vi "main.vi"() -> ()   [LabVIEW 2023]
uses:
  #typedef_typ.ctl
  #typedef_state.ctl
  #typdef_data.ctl
  08a89311-3c14-40fd-979e-0ee36f0e0fa9.vi
  <vilib>/Array/Sort 2D Array - Pop Stack.vi
  <vilib>/Array/Sort 2D Array - Push Stack.vi
  <vilib>/Utility/file.llb/Read Delimited Spreadsheet (string).vi
  <vilib>/Utility/file.llb/Write Delimited Spreadsheet (string).vi
panel:
  in  "Producent":string
  in  "Nazwa":string
  in  "Numer":string
  in  "Sort":bool
  in  "Add":bool
  in  "Delete":bool
  in  "Search":bool
  in  "Show":bool
  in  "Stop Button":bool
  in  "Produkt":string
  out "Wyswietlacz":string[][](array[string])
  in  "Type":T1
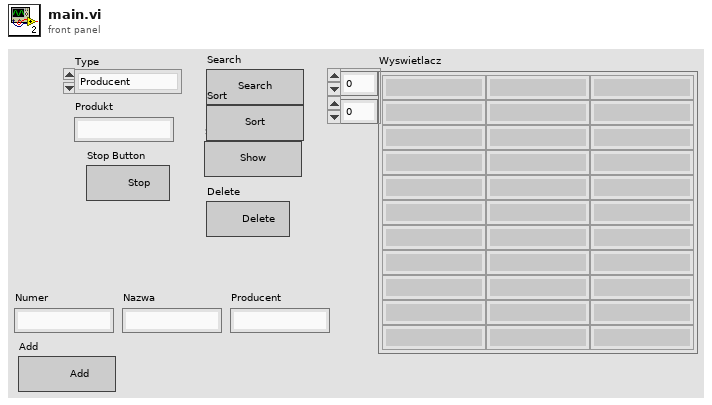
[diagram p1: front panel]
types:
  T1 = typedef "#typedef_typ.ctl" = enum16{"Producent", "Nazwa produktu", "Numer produktu"}
  T2 = typedef "#typedef_state.ctl" = enum16{"Aplication error", "Show", "Idle", "Open", "Search", "Add", "Delete", "Sort", "Exit"}
  T3 = typedef "#typdef_data.ctl" = cluster{"Type":enum16{"Producent", "Nazwa produktu", "Numer produktu"}, "Dane":string[][], "Produkt":string}
  T4 = enum16{"Producent", "Nazwa produktu", "Numer produktu"}
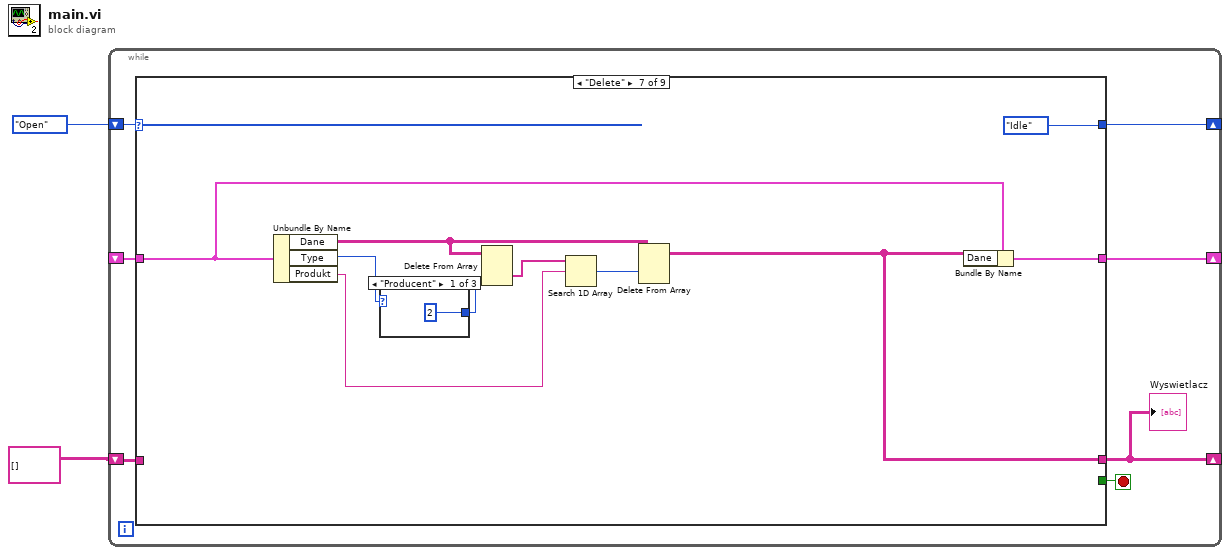
[diagram p0: block diagram]
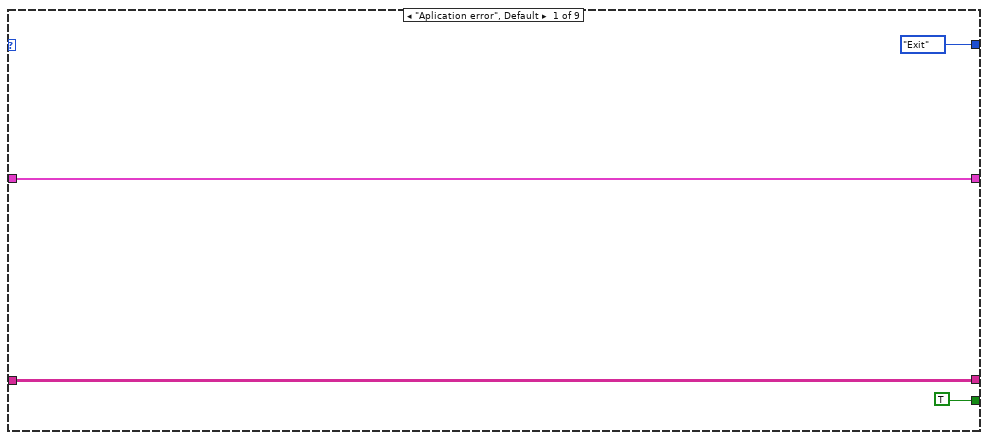
[diagram p2: hidden frame]
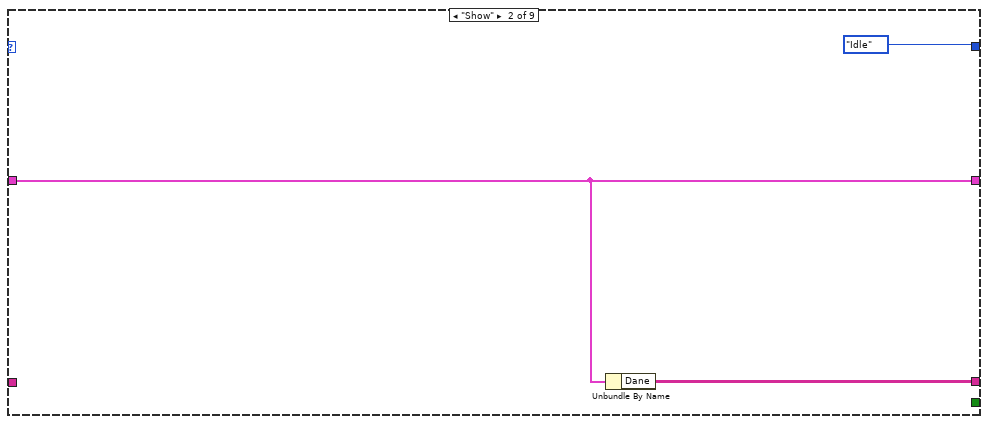
[diagram p3: hidden frame]
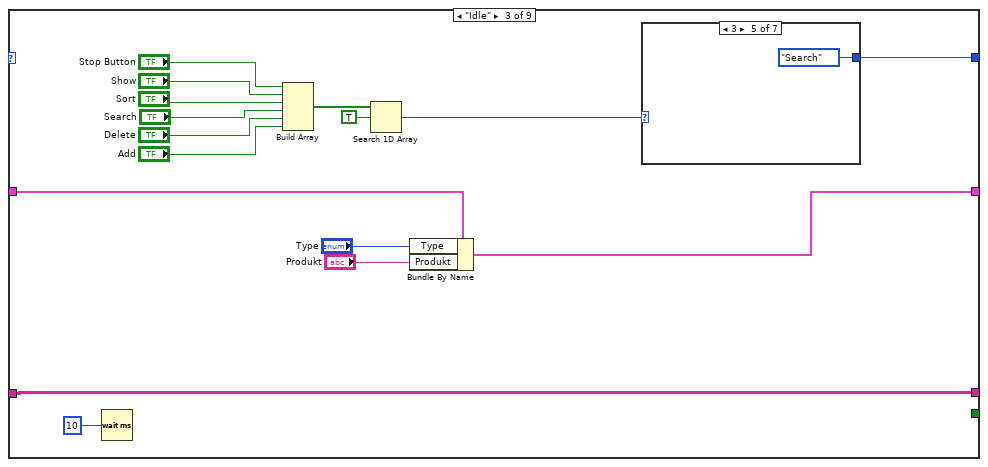
[diagram p4: hidden frame]
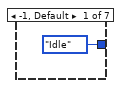
[diagram p5: hidden frame]
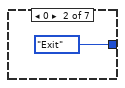
[diagram p6: hidden frame]
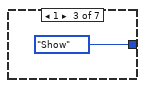
[diagram p7: hidden frame]
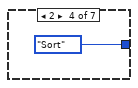
[diagram p8: hidden frame]
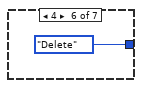
[diagram p9: hidden frame]
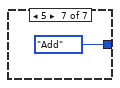
[diagram p10: hidden frame]
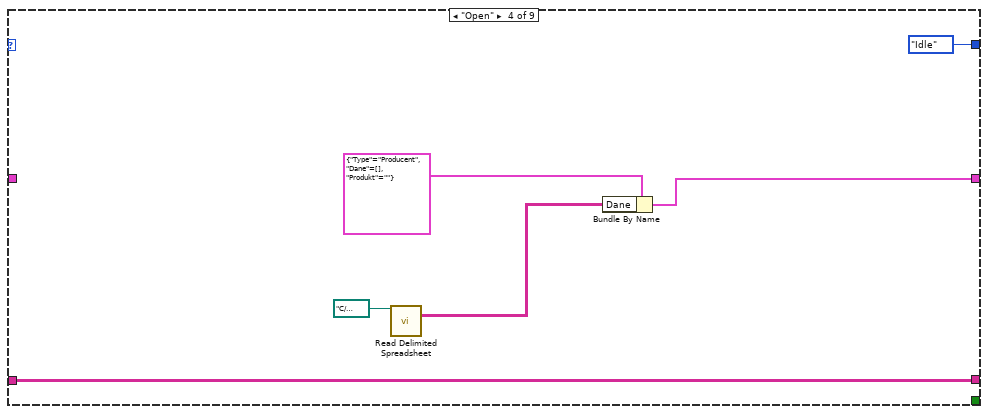
[diagram p11: hidden frame]
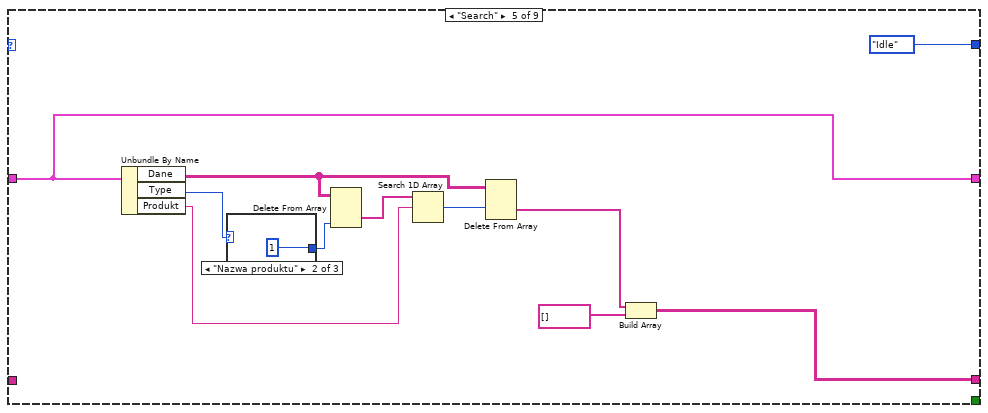
[diagram p12: hidden frame]
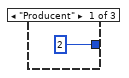
[diagram p13: hidden frame]
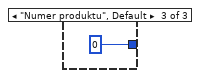
[diagram p14: hidden frame]
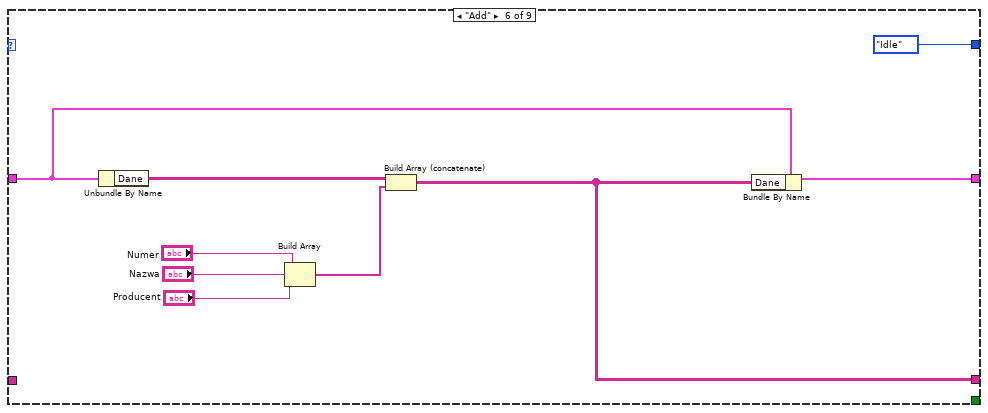
[diagram p15: hidden frame]
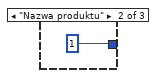
[diagram p16: hidden frame]
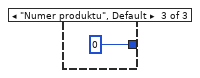
[diagram p17: hidden frame]
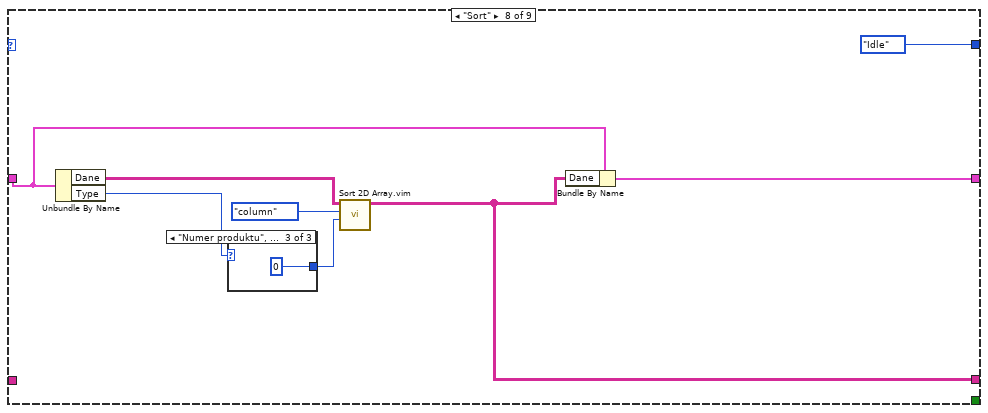
[diagram p18: hidden frame]
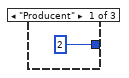
[diagram p19: hidden frame]
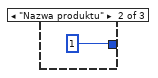
[diagram p20: hidden frame]
diagram:
  n1 = while {
    shift-right: [w8] -> _
    shift-left: #typedef_state."Open" ("State") -> [w9]
    shift-right: [w7] -> _
    shift-left: _ -> [w6]
    shift-right: [w3] -> _
    shift-left: string[][] [] ("Dane") -> [w4]
    stop <- w5 stop-if-true
    n2 = case shown="\"Delete\"" w9 {
      tunnel: [#typedef_state."Exit" ("State") #typedef_state."Idle" ("State") w17 #typedef_state."Idle" ("State") #typedef_state."Idle" ("State") #typedef_state."Idle" ("State") #typedef_state."Idle" ("State") #typedef_state."Idle" ("State") #typedef_state."Exit" ("State")] -> w8
      tunnel: [w12 w16 w28 w42 w50 w61 w73 w82 w96] -> w7
      tunnel: w6 -> [w12 w16 w32 _ w50 w63 w74 w83 w96]
      tunnel: [TRUE _ _ _ _ _ _ _ TRUE] -> w5
      tunnel: [w10 w15 w29 w40 w51 w62 w75 w84 w93] -> w3
      tunnel: w4 -> [w10 _ w29 w40 _ _ _ _ w93]
      frame "Aplication error", Default {
      }
      frame "Show" {
        n3 = Unbundle By Name(w16) -> ("Dane"=w15:string[][])
      }
      frame "Idle" {
        n4 = Wait (ms)(milliseconds to wait=u32 10) -> ()  [unwired: 1 out]
        n5 = Build Array("Stop Button", "Show", "Sort", "Search", "Delete", "Add") -> (w21:bool[])
        n6 = Search 1D Array(1D array=w21, element=TRUE) -> (index of element=w19:i32)  [unwired: 1 in]
        n7 = Bundle By Name(cluster=w32, "Type"="Type", "Produkt"="Produkt") -> (w28:T3)
        n8 = case shown="3" w19 {
          tunnel: [#typedef_state."Idle" ("State") #typedef_state."Exit" ("State") #typedef_state."Show" ("State") #typedef_state."Sort" ("State") #typedef_state."Search" ("State") #typedef_state."Delete" ("State") #typedef_state."Add" ("State")] -> w17
          frame -1, Default {
          }
          frame 0 {
          }
          frame 1 {
          }
          frame 2 {
          }
          frame 3 {
          }
          frame 4 {
          }
          frame 5 {
          }
        }
      }
      frame "Open" {
        n9 = call-poly <vilib>:"Read Delimited Spreadsheet.vi"("file path (dialog if empty)"=path "C:/Users/Python/Desktop/LabView Zadania/Wyklad - Maj/Zestaw 7 - State Machine/Zad2/baza.csv") -> ("all rows"=w41:string[][])  [unwired: 9 in, 5 out]
        n10 = Bundle By Name(cluster=T3 {"Type"=enum."Producent", "Dane"=[], "Produkt"=""} ("Data"), "Dane"=w41) -> (w42:T3)
      }
      frame "Search" {
        n11 = Unbundle By Name(w50) -> ("Dane"=w48:string[][], "Type"=w56:T4, "Produkt"=w55:string)
        n12 = case shown="\"Nazwa produktu\"" w56 {
          tunnel: [2 1 0] -> w47
          frame "Producent" {
          }
          frame "Nazwa produktu" {
          }
          frame "Numer produktu", Default {
          }
        }
        n13 = Delete From Array(array=w48, index (col)=w47) -> (deleted portion=w46:string[])  [unwired: 2 in, 1 out]
        n14 = Search 1D Array(1D array=w46, element=w55) -> (index of element=w54:i32)  [unwired: 1 in]
        n15 = Delete From Array(array=w48, index (row)=w54) -> (deleted portion=w53:string[])  [unwired: 2 in, 1 out]
        n16 = Build Array(w53, string[] [] ("element")) -> (w51:string[][])
      }
      frame "Add" {
        n17 = Unbundle By Name(w63) -> ("Dane"=w64:string[][])
        n18 = Build Array("Numer", "Nazwa", "Producent") -> (w65:string[])
        n19 = Build Array (concatenate)(w64, w65) -> (w62:string[][])
        n20 = Bundle By Name(cluster=w63, "Dane"=w62) -> (w61:T3)
      }
      frame "Delete" {
        n21 = Unbundle By Name(w74) -> ("Dane"=w71:string[][], "Type"=w78:T4, "Produkt"=w77:string)
        n22 = case shown="\"Producent\"" w78 {
          tunnel: [2 1 0] -> w70
          frame "Producent" {
          }
          frame "Nazwa produktu" {
          }
          frame "Numer produktu", Default {
          }
        }
        n23 = Delete From Array(array=w71, index (col)=w70) -> (deleted portion=w69:string[])  [unwired: 2 in, 1 out]
        n24 = Search 1D Array(1D array=w69, element=w77) -> (index of element=w76:i32)  [unwired: 1 in]
        n25 = Delete From Array(array=w71, index (row)=w76) -> (array with subset deleted=w75:string[][])  [unwired: 2 in, 1 out]
        n26 = Bundle By Name(cluster=w74, "Dane"=w75) -> (w73:T3)
      }
      frame "Sort" {
        n27 = Unbundle By Name(w83) -> ("Dane"=w87:string[][], "Type"=w86:T4)
        n28 = case shown="\"Numer produktu\", Default" w86 {
          tunnel: [2 1 0] -> w85
          frame "Producent" {
          }
          frame "Nazwa produktu" {
          }
          frame "Numer produktu", Default {
          }
        }
        n29 = call "Sort 2D Array.vim"("index"=w85, "dimension to index (column)"=enum16{"column", "row"}."column", "2D array"=w87) -> ("sorted 2D array"=w84:string[][])  [unwired: 7 in, 1 out]
        n30 = Bundle By Name(cluster=w83, "Dane"=w84) -> (w82:T3)
      }
      frame "Exit" {
        n31 = Unbundle By Name(w96) -> ("Dane"=w97:string[][])
        n32 = call-poly <vilib>:"Write Delimited Spreadsheet.vi"("file path (dialog if empty)"=path "C:/Users/Python/Desktop/LabView Zadania/Wyklad - Maj/Zestaw 7 - State Machine/Zad2/baza.csv", "2D data"=w97) -> ()  [unwired: 12 in, 2 out]
      }
    }
    "Wyswietlacz" <- w3
  }
